vi "change table color.vi"(11 "MulticolumnListbox输入":refnum<vi>) -> ()   [LabVIEW 2016]
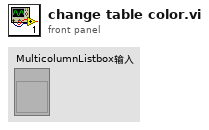
[diagram p1: front panel]
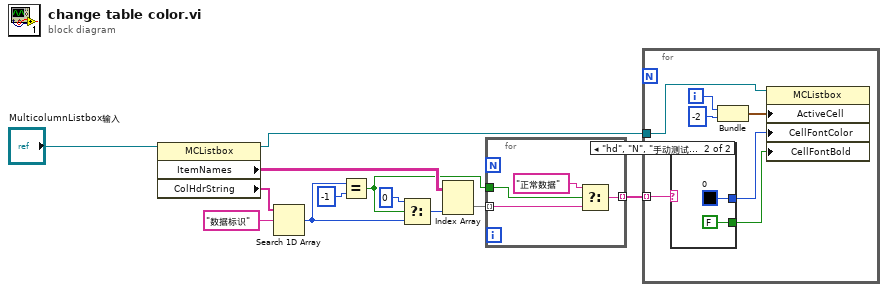
[diagram p0: block diagram]
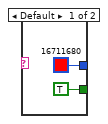
[diagram p2: hidden frame]
diagram:
  n1 = property class="MCListbox"(reference="MulticolumnListbox输入") -> (reference out=w12:refnum<vi>, "ItemNames"=w11:string[][], "ColHdrString"=w9:string[])  [unwired: 1 in, 1 out]
  n2 = Search 1D Array(1D array=w9, element="数据标识" ("元素")) -> (index of element=w6:i32)  [unwired: 1 in]
  n3 = Equal?(x=w6, y=-1) -> (x = y?=w2:bool)
  n4 = Select(t=0, s=w2, f=w6) -> (s? t:f=w4:i32)
  n5 = Index Array(array=w11, index (col)=w4) -> (element=w3:string[])  [unwired: 1 in]
  n6 = for {
    tunnel: w3 -> [w14] mode=indexing
    tunnel: w2 -> [w16]
    tunnel: [w13] -> w1 mode=indexing
    n7 = Select(t="正常数据", s=w16, f=w14) -> (s? t:f=w13:string)
  }
  n8 = for {
    tunnel: w1 -> [w23] mode=indexing
    tunnel: w12 -> [w22]
    i -> [w19]
    n9 = case shown="\"hd\", \"N\", \"手动测试数据\", \"正常数据\"" w23 {
      tunnel: [TRUE FALSE] -> w20
      tunnel: [u32 16711680 u32 0] -> w21
      frame Default {
      }
      frame "hd", "N", "手动测试数据", "正常数据" {
      }
    }
    n10 = Bundle(w19, -2) -> (w17:cluster{i32, i32})  [unwired: 1 in]
    n11 = property class="MCListbox"(reference=w22, "ActiveCell"=w17, "CellFontColor"=w21, "CellFontBold"=w20) -> ()  [unwired: 1 in, 2 out]
  }
